vi "Station_meteo.vi"() -> ()   [LabVIEW 2018]
uses:
  <vilib>/Instr/_visa.llb/VISA Configure Serial Port (Instr).vi
panel:
  out "Moyenne Temp":dbl
  out "Moyenne Press":dbl
  out "Maximum Humi":dbl
  out "Maximum Temp":dbl
  in  "Minimum Humi":dbl
  in  "Minimum Press":dbl
  in  "Minimum Temp":dbl
  out "Moyenne Humi":dbl
  out "Maximum Press":dbl
  out "Ligne":string
  out "Humidity":dbl
  out "Pressure":dbl
  out "Temperature":dbl
  in  "Pause":bool
  out "Humidity":dbl(graph)
  out "Pressure":dbl(graph)
  out "Temperature":dbl(graph)
  out "Chaîne":string
  in  "stop":bool
  in  "Nom de ressource VISA":refnum<visa-resource-name>
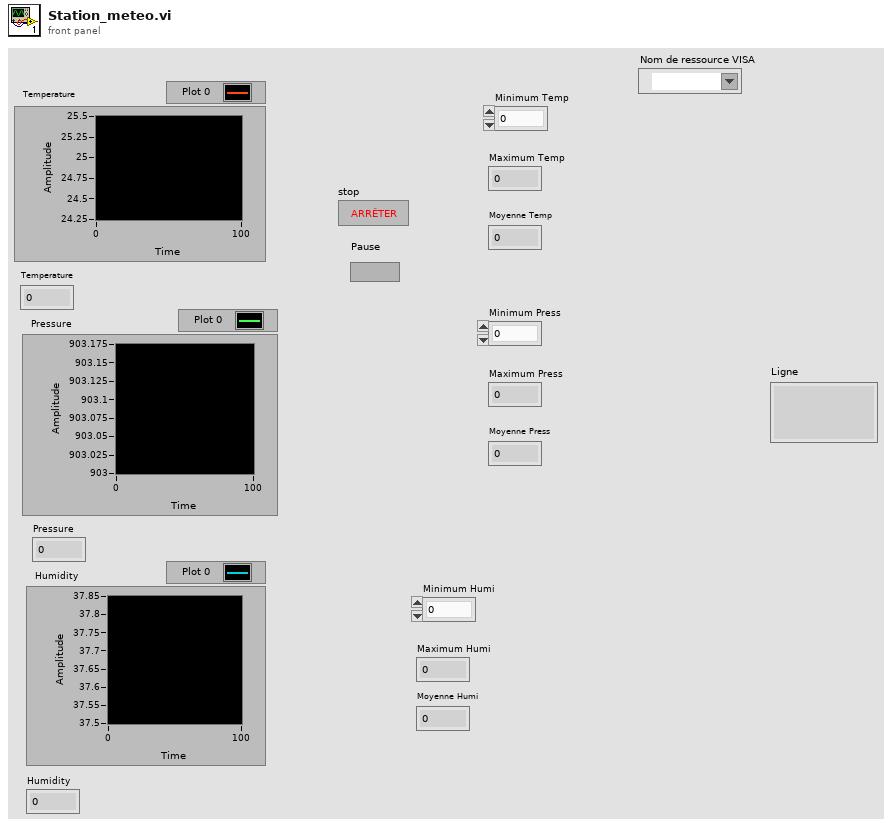
[diagram p1: front panel]
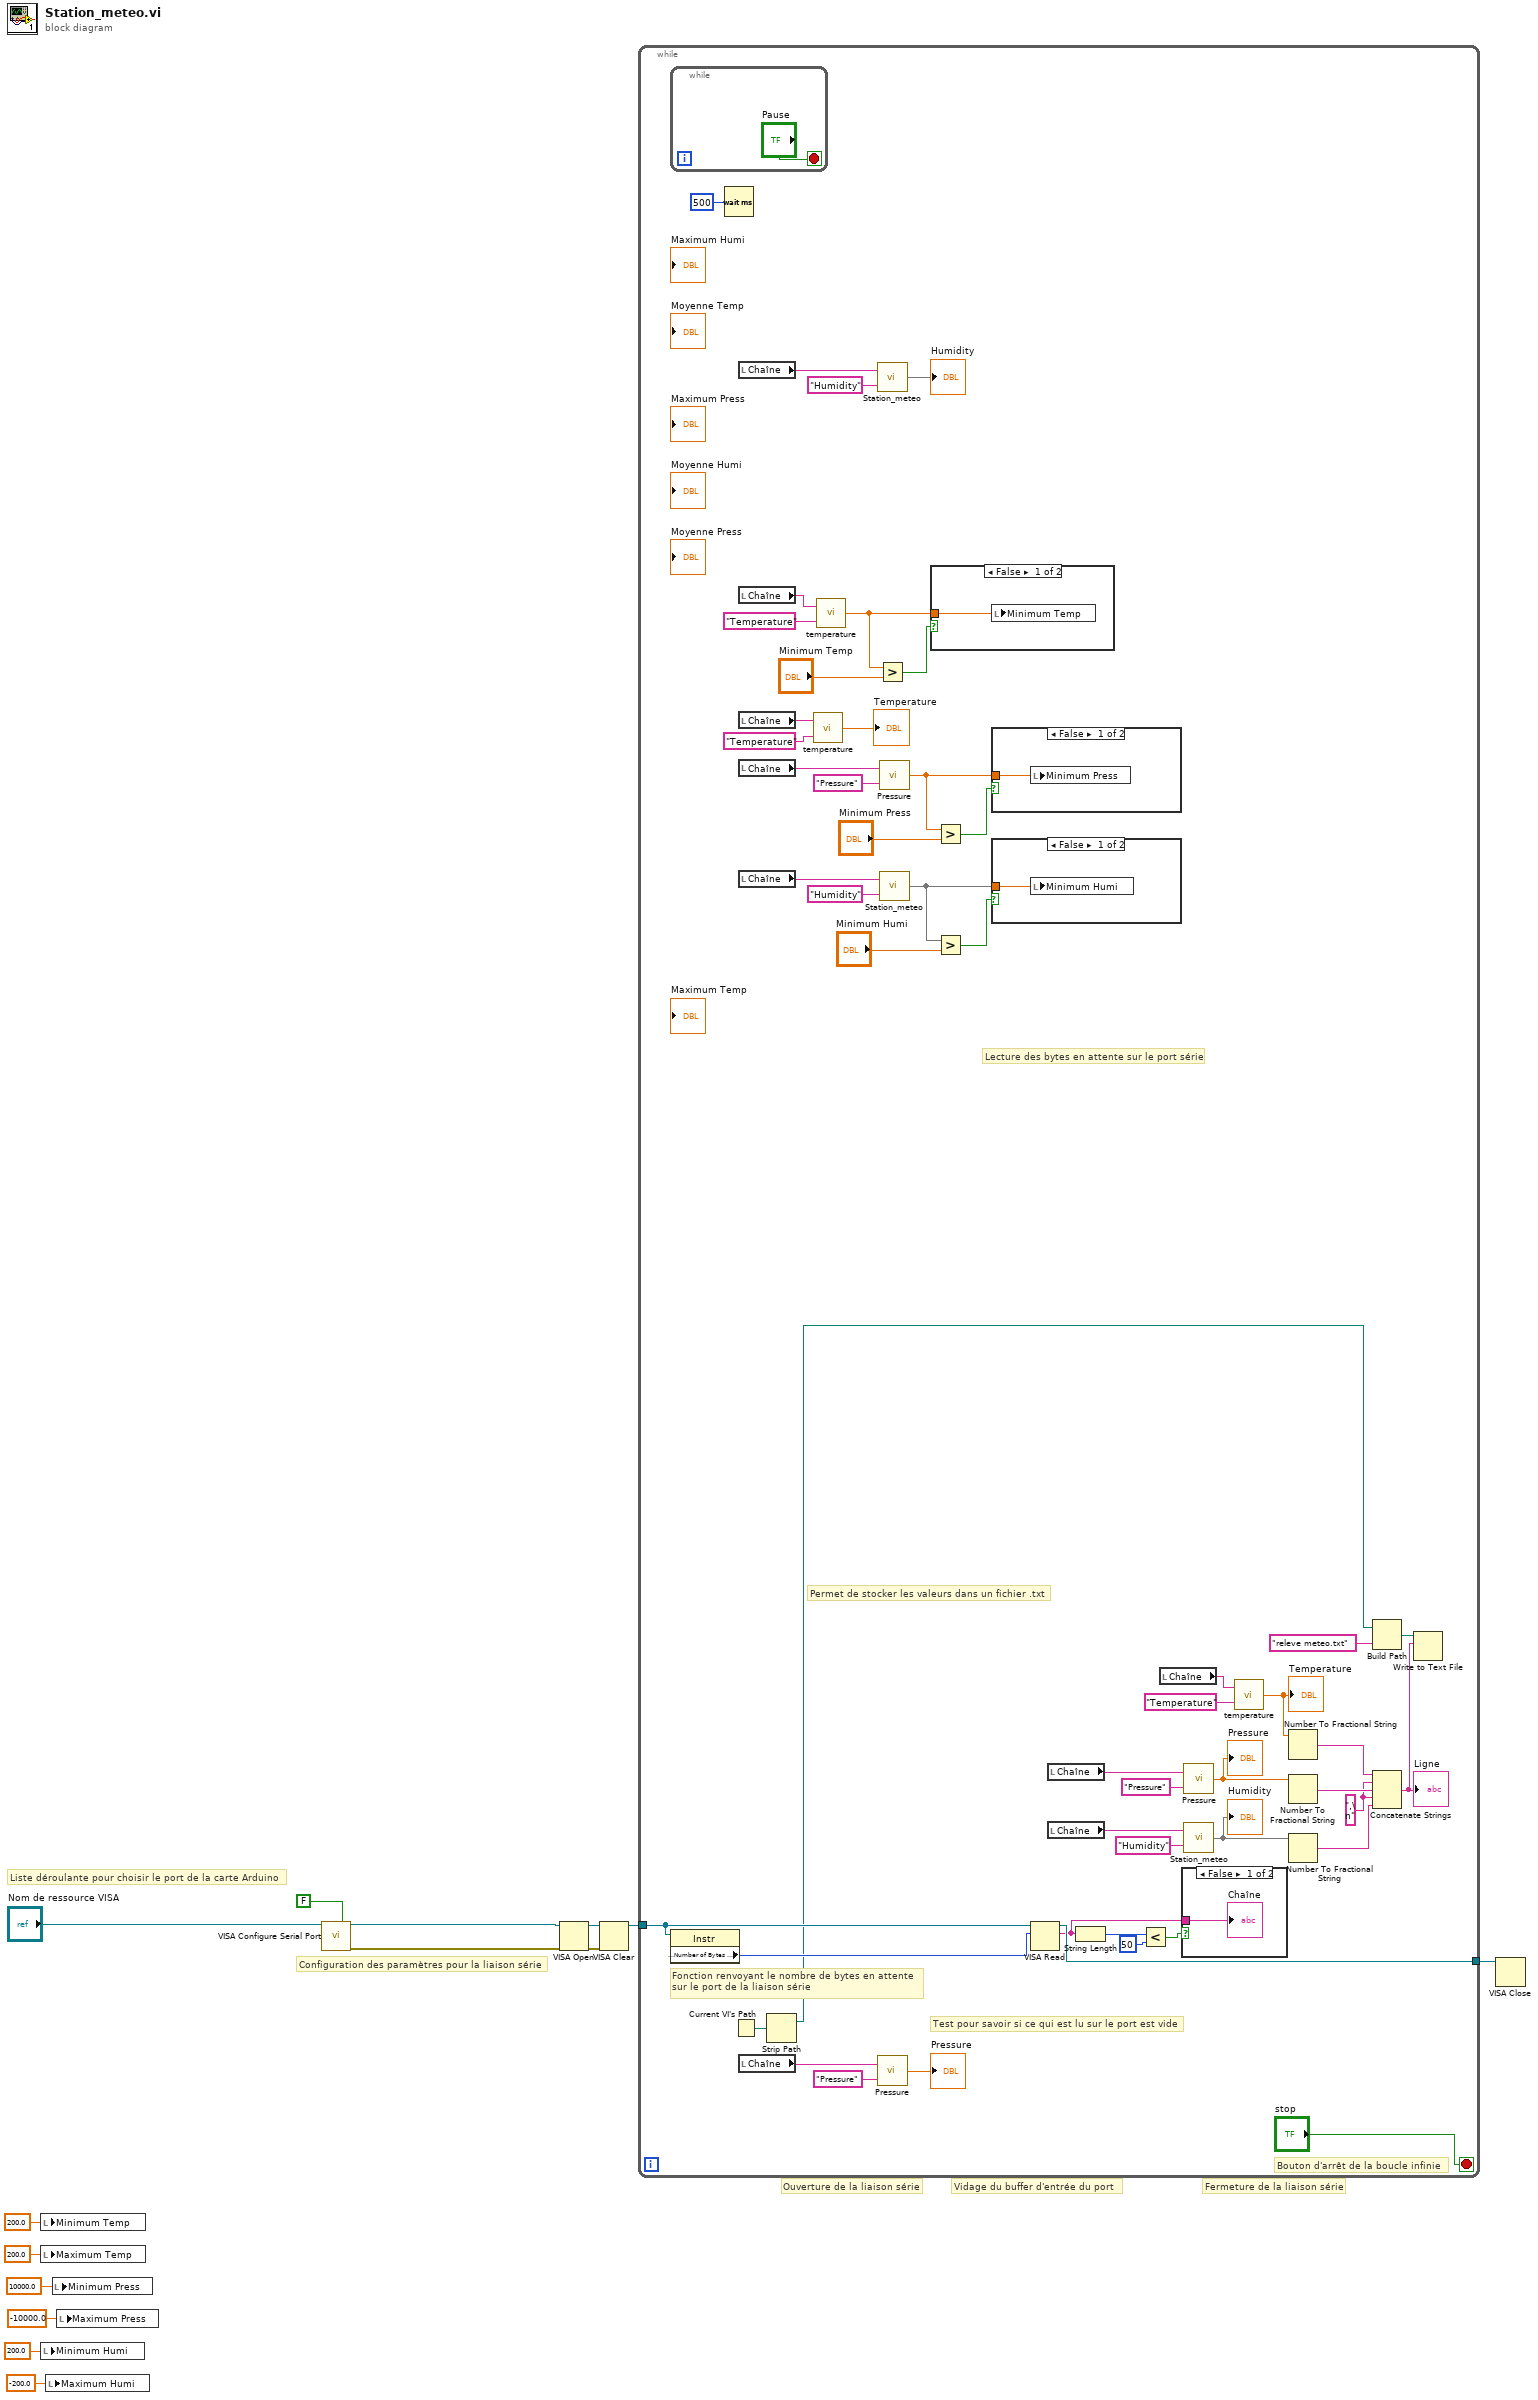
[diagram p0: block diagram]
diagram:
  # "Vidage du buffer d'entrée du port"
  # "Ouverture de la liaison série"
  # "Configuration des paramètres pour la liaison série"
  # "Liste déroulante pour choisir le port de la carte Arduino"
  # "Fermeture de la liaison série"
  n1 = local write "Minimum Temp"(200.0 ("Minimum")) -> ()
  n2 = local write "Maximum Temp"(200.0 ("Minimum")) -> ()
  n3 = local write "Minimum Humi"(200.0 ("Minimum")) -> ()
  n4 = local write "Maximum Humi"(-200.0 ("Minimum")) -> ()
  n5 = local write "Minimum Press"(10000.0 ("Minimum")) -> ()
  n6 = local write "Maximum Press"(-10000.0 ("Minimum")) -> ()
  n7 = call-poly "VISA Configure Serial Port"("VISA resource name"="Nom de ressource VISA", "Enable Termination\nChar (T)"=FALSE ("Enable Termination\nChar (T)")) -> ("VISA resource name out"=w11:refnum<visa-resource-name>, "error out"=w9:errorcluster)  [unwired: 12 in]
  n8 = VISA Open(error in (no error)=w9, VISA resource name=w11) -> (VISA resource name=w13:refnum<visa-resource-name>, error out=w8:errorcluster)  [unwired: 3 in]
  n9 = VISA Clear(VISA resource name=w13, error in (no error)=w8) -> (VISA resource name out=w12:refnum<visa-resource-name>)  [unwired: 1 out]
  n10 = while {
    tunnel: w12 -> [w64]
    tunnel: [w62] -> w7
    stop <- "stop" stop-if-true
    w34 = ",\n" ("string")
    # "Permet de stocker les valeurs dans un fichier .txt"
    # "Lecture des bytes en attente sur le port série"
    # "Fonction renvoyant le nombre de bytes en attente\nsur le port de la liaison série"
    # "Test pour savoir si ce qui est lu sur le port est vide"
    # "Bouton d'arrêt de la boucle infinie"
    n11 = while {
      stop <- "Pause" stop-if-true
    }
    n12 = property class="Instr"(reference=w64) -> ("Serial Settings:Number of Bytes at Serial Port"=w63:u32)  [unwired: 1 in, 2 out]
    n13 = Wait (ms)(milliseconds to wait=u32 500 ("attente (ms)")) -> ()  [unwired: 1 out]
    n14 = Current VI's Path() -> (path=w39:path)
    n15 = local read "Chaîne"() -> (w53:string)
    n16 = local read "Chaîne"() -> (w32:string)
    n17 = local read "Chaîne"() -> (w55:string)
    n18 = local read "Chaîne"() -> (w23:string)
    n19 = local read "Chaîne"() -> (w17:string)
    n20 = local read "Chaîne"() -> (w54:string)
    n21 = Strip Path(path=w39) -> (stripped path=w38:path)  [unwired: 1 out]
    n22 = call "temperature.vi"("Variable name"="Temperature", "Chaîne"=w55) -> ("Numeric"=→"Temperature":dbl)
    n23 = call "temperature.vi"("Variable name"="Temperature", "Chaîne"=w32) -> ("Numeric"=w29:dbl)
    n24 = call "Station_meteo.vi"(1:"Humidity", 2:w53) -> (0:→"Humidity")
    n25 = Greater?(x=w29, y="Minimum Temp") -> (0:w31:bool)
    n26 = call "Pressure.vi"("Variable name"="Pressure", "Chaîne"=w54) -> ("Numeric"=→"Pressure":dbl)
    n27 = call "Pressure.vi"("Variable name"="Pressure", "Chaîne"=w23) -> ("Numeric"=w20:dbl)
    n28 = call "Station_meteo.vi"(1:"Humidity", 2:w17) -> (0:w15)
    n29 = case shown="False" w31 {
      tunnel: w29 -> [w68 _]
      frame False {
        n30 = local write "Minimum Temp"(w68) -> ()
      }
      frame True {
      }
    }
    n31 = Greater?(x=w20, y="Minimum Press") -> (0:w21:bool)
    n32 = Greater?(x=w15, y="Minimum Humi") -> (0:w18:bool)
    n33 = case shown="False" w21 {
      tunnel: w20 -> [w67 _]
      frame False {
        n34 = local write "Minimum Press"(w67) -> ()
      }
      frame True {
      }
    }
    n35 = case shown="False" w18 {
      tunnel: w15 -> [w66 _]
      frame False {
        n36 = local write "Minimum Humi"(w66) -> ()
      }
      frame True {
      }
    }
    n37 = VISA Read(VISA resource name=w64, byte count=w63) -> (VISA resource name out=w62:refnum<visa-resource-name>, read buffer=w28:string)  [unwired: 1 in, 2 out]
    n38 = local read "Chaîne"() -> (w49:string)
    n39 = local read "Chaîne"() -> (w47:string)
    n40 = String Length(string=w28) -> (length=w27:i32)
    n41 = Less?(x=w27, y=50) -> (x < y?=w25:bool)
    n42 = local read "Chaîne"() -> (w50:string)
    n43 = case shown="False" w25 {
      tunnel: w28 -> [w70 _]
      frame False {
        "Chaîne" <- w70
      }
      frame True {
      }
    }
    n44 = call "Pressure.vi"("Variable name"="Pressure", "Chaîne"=w49) -> ("Numeric"=w42:dbl)
    "Pressure" <- w42
    n45 = call "Station_meteo.vi"(1:"Humidity", 2:w47) -> (0:w43)
    "Humidity" <- w43
    n46 = call "temperature.vi"("Variable name"="Temperature", "Chaîne"=w50) -> ("Numeric"=w45:dbl)
    "Temperature" <- w45
    n47 = Number To Fractional String(number=w45) -> (F-format string=w44:string)  [unwired: 3 in]
    n48 = Number To Fractional String(number=w42) -> (F-format string=w41:string)  [unwired: 3 in]
    n49 = Number To Fractional String(number=w43) -> (F-format string=w40:string)  [unwired: 3 in]
    n50 = Build Path(base path=w38, name or relative path="releve meteo.txt") -> (appended path=w36:path)
    n51 = Concatenate Strings(w44, w34, w41, w34, w40) -> (w35:string)
    "Ligne" <- w35
    n52 = Write to Text File(file (use dialog)=w36, text=w35) -> ()  [unwired: 2 in, 3 out]
  }
  n53 = VISA Close(VISA resource name=w7) -> ()  [unwired: 1 in, 1 out]
